vi "Validate Get Connections Outputs.vi"(4 "pin type":T1, 6 "site":i32, 8 "error in":errorcluster, 9 "instrument type id":string, 10 "pin or relay names":string[](array[string]), 11 "pin or relay names found":string[](array[string])) -> (0 "error out":errorcluster)   [LabVIEW 2020, in "Plug-In SDK Session Management V1 API.lvlib" / "Session Reservation.lvclass"]
uses:
  Session Reservation.lvclass
  a25400be-0e32-497d-9f89-976053e83216.vi
  Pin Type.ctl
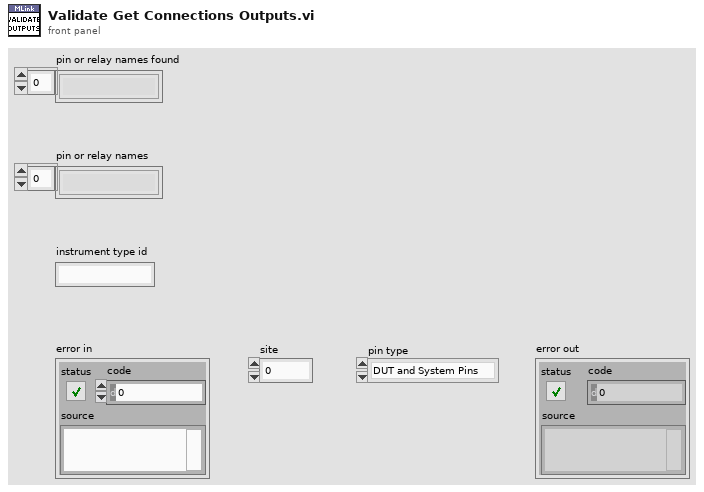
[diagram p1: front panel]
types:
  T1 = typedef "Plug-In SDK Session Management V1 API.lvlib/Session Reservation.lvclass/Pin Type.ctl" = enum16{"DUT and System Pins", "System Pins"}
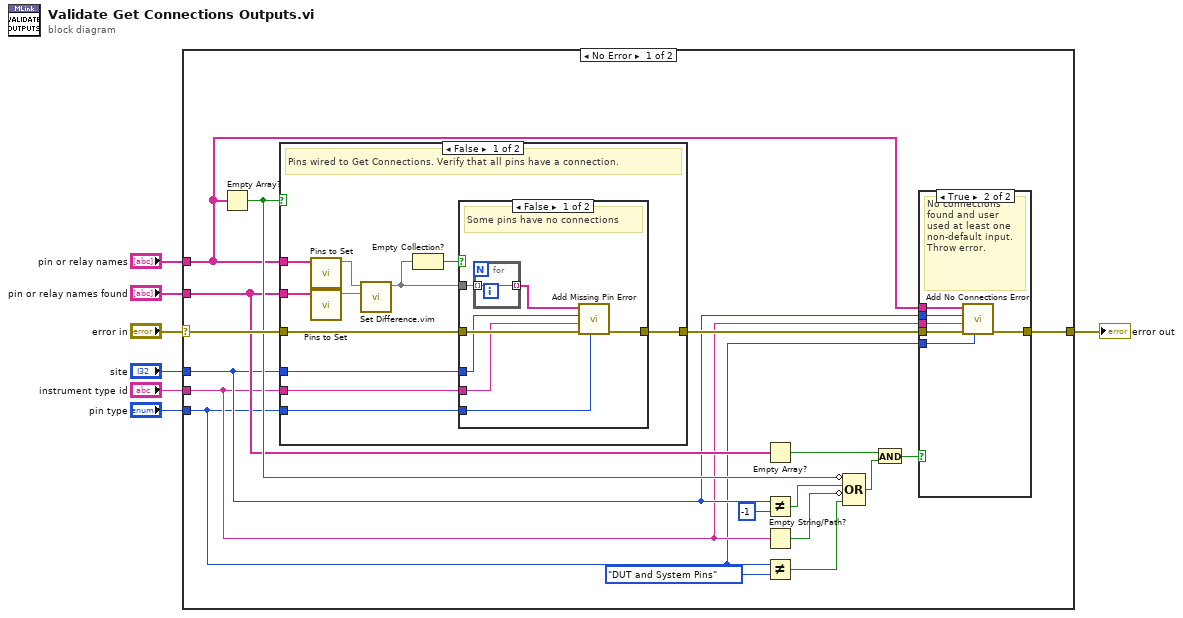
[diagram p0: block diagram]
diagram:
  n1 = case shown="No Error" "error in" {
    selector: "error in" -> [w24 w53]
    tunnel: "pin or relay names" -> [w13 _]
    tunnel: "site" -> [w12 _]
    tunnel: "instrument type id" -> [w11 _]
    tunnel: [w19 w53] -> w2
    tunnel: "pin or relay names found" -> [w16 _]
    tunnel: "pin type" -> [w8 _]
    frame No Error {
      n2 = Empty Array?(array=w13) -> (empty?=w18:bool)
      n3 = case shown="False" w18 {
        tunnel: w16 -> [w31 _]
        tunnel: w13 -> [w30 _]
        tunnel: w24 -> [w29 w45]
        tunnel: [w28 w45] -> w20
        tunnel: w12 -> [w27 _]
        tunnel: w11 -> [w26 _]
        tunnel: w8 -> [w25 _]
        frame False {
          # "Pins wired to Get Connections. Verify that all pins have a connection."
          n4 = call "Pins to Set.vi"("pin or relay names array"=w30) -> ("pin or relay name set"=w34:set{string})  [unwired: 10 in]
          n5 = call "Pins to Set.vi"("pin or relay names array"=w31) -> ("pin or relay name set"=w35:set{string})  [unwired: 10 in]
          n6 = call "Set Difference.vim"("set 2"=w35, "set 1"=w34) -> ("difference"=w33:set{string})  [unwired: 9 in]
          n7 = Empty Collection?(1:w33) -> (0:w32:bool)
          n8 = case shown="False" w32 {
            tunnel: w29 -> [w41 w44]
            tunnel: [w40 w44] -> w28
            tunnel: w33 -> [w42 _]
            tunnel: w27 -> [w38 _]
            tunnel: w26 -> [w37 _]
            tunnel: w25 -> [w36 _]
            frame False {
              # "Some pins have no connections"
              n9 = for {
                tunnel: w42 -> [w43] mode=indexing
                tunnel: [w43] -> w39 mode=indexing
              }
              n10 = call "Add Missing Pin Error.vi"("pin type"=w36, "error in"=w41, "instrument type id"=w37, "site"=w38, "missing pin or relay names"=w39) -> ("error out"=w40:errorcluster)  [unwired: 6 in]
            }
            frame True {
              # "All pins have connections"
            }
          }
        }
        frame True {
          # "Pins not wired to Get Connections. No verification required."
        }
      }
      n11 = Empty Array?(array=w16) -> (empty?=w15:bool)
      n12 = Not Equal?(x=w12, y=-1) -> (x != y?=w14:bool)
      n13 = Empty String/Path?(string/path=w11) -> (empty?=w21:bool)
      n14 = Not Equal?(x=w8, y=Pin_Type."DUT and System Pins") -> (x != y?=w9:bool)
      n15 = Compound Arithmetic op=OR(invert w18, w14, invert w21, w9) -> (w23:bool)
      n16 = And(x=w15, y=w23) -> (x .and. y?=w17:bool)
      n17 = case shown="True" w17 {
        tunnel: w20 -> [w46 w52]
        tunnel: [w46 w51] -> w19
        tunnel: w13 -> [_ w50]
        tunnel: w12 -> [_ w49]
        tunnel: w11 -> [_ w48]
        tunnel: w8 -> [_ w47]
        frame False {
          # "No connections found, but only default inputs specified. No error."
        }
        frame True {
          # "No connections found and user used at least one non-default input. Throw error."
          n18 = call "Add No Connections Error.vi"("pin type"=w47, "error in"=w52, "instrument type id"=w48, "site"=w49, "pin or relay names"=w50) -> ("error out"=w51:errorcluster)  [unwired: 6 in]
        }
      }
    }
    frame Error {
    }
  }
  "error out" <- w2
